vi "Get Boolean.vi"(8 "error in (no error)":errorcluster, 9 "Data Type (default value)":bool, 10 "Offset":i32, 11 "JSON":string) -> (0 "error out":errorcluster, 1 "Boolean":bool, 2 "Offset past match":i32)   [LabVIEW 2024, in "JSONtext.lvlib"]
uses:
  JSONtext.lvlib
  Error Cluster From Error Code.vi
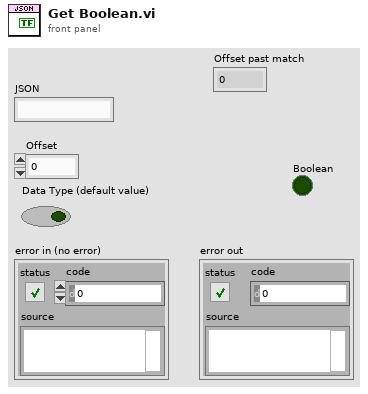
[diagram p1: front panel]
types:
  T1 = typedef "JSONtext.lvlib/Parsing State.ctl" = enum16{"Parser Error", "Object", "Array", "String", "Number/Other", "Leading Whitespace", "Object end", "Array end", "Value end"}
  T2 = typedef "JSONtext.lvlib/JSON Value Type.ctl" = enum16{"Not a JSON Value", "JSON Object", "JSON Array", "String", "Number", "true", "false", "null"}
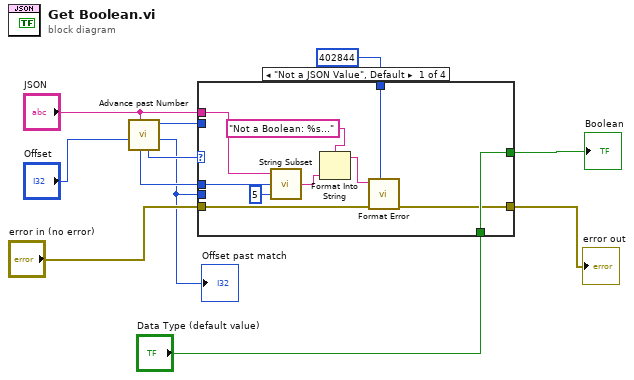
[diagram p0: block diagram]
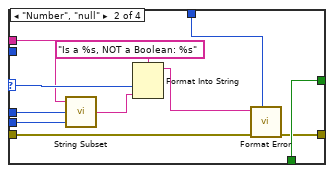
[diagram p2: hidden frame]
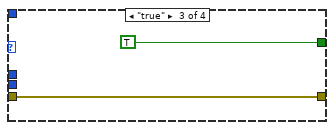
[diagram p3: hidden frame]
diagram:
  n1 = call "Advance past Number.vi"("JSON"="JSON", "Offset (0)"="Offset") -> ("Offset past match"=w4:i32, "Parser State"=w2:T1, "JSON Value Type"=w7:T2, "Value start out"=w5:i32)  [unwired: 5 in, 1 out]
  "Offset past match" <- w4
  n2 = case shown="\"Not a JSON Value\", Default" w7 {
    selector: w7 -> [_ w29 _ _]
    tunnel: [w21 w32 TRUE _] -> w11
    tunnel: [w20 w31 w33 w35] -> w10
    tunnel: "error in (no error)" -> [w19 w30 w33 w35]
    tunnel: "Data Type (default value)" -> [w21 w32 _ _]
    tunnel: w5 -> [w17 w26 _ _]
    tunnel: w4 -> [_ w25 _ _]
    tunnel: "JSON" -> [w18 w24 _ _]
    tunnel: w2 -> [_ _ _ _]
    tunnel: 402844 ("error code (402842)") -> [w12 w22 _ _]
    frame "Not a JSON Value", Default {
      n3 = call "String Subset.vi"("Offset past End"=5, "Start offset"=w17, "JSON"=w18) -> ("substring"=w14:string)  [unwired: 2 in]
      n4 = Format Into String(format string="Not a Boolean: %s...", w14) -> (resulting string=w13:string)  [unwired: 2 in, 1 out]
      n5 = call "Format Error.vi"("error code (402842)"=w12, "error in (no error)"=w19, "error message"=w13) -> ("error out"=w20:errorcluster)  [unwired: 8 in]
    }
    frame "Number", "null" {
      n6 = call "String Subset.vi"("Offset past End"=w25, "Start offset"=w26, "JSON"=w24) -> ("substring"=w23:string)  [unwired: 2 in]
      n7 = Format Into String(format string="Is a %s, NOT a Boolean: %s", w29, w23) -> (resulting string=w27:string)  [unwired: 2 in, 1 out]
      n8 = call "Format Error.vi"("error code (402842)"=w22, "error in (no error)"=w30, "error message"=w27) -> ("error out"=w31:errorcluster)  [unwired: 8 in]
    }
    frame "true" {
    }
    frame "false" {
    }
  }
  "error out" <- w10
  "Boolean" <- w11
